vi "VISA LoopRead.vi"(8 "error in (no error)":errorcluster, 9 "byte count (350000)":u32=350000, 11 "VISA resource name":refnum<visa-resource-name>="GPIB0::4::INSTR") -> (0 "error out":errorcluster={"status"=FALSE, "code"=1073676294, "source"="VISA Read in CSA Measure.vi"}, 1 "Total Buffer":string, 3 "dup VISA resource name":refnum<visa-resource-name>="GPIB0::4::INSTR")   [LabVIEW 2011]
panel:
  out "Loops Performed":i32
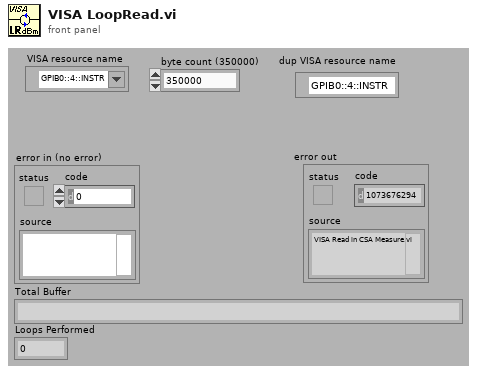
[diagram p1: front panel]
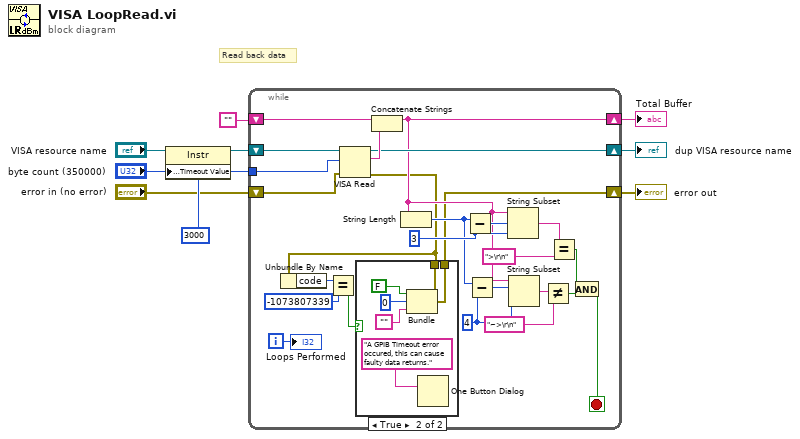
[diagram p0: block diagram]
diagram:
  # "Read back data"
  n1 = property class="Instr"(reference="VISA resource name", "General Settings:Timeout Value"=u32 3000) -> (reference out=w4:refnum<visa-resource-name>)  [unwired: 1 in, 1 out]
  n2 = while {
    shift-left: "error in (no error)" -> [w11]
    shift-right: [w17] -> w6
    shift-left: w4 -> [w10]
    shift-right: [w31] -> w7
    shift-left: "" -> [w32]
    shift-right: [w21] -> w8
    tunnel: "byte count (350000)" -> [w34]
    i -> [w15]
    stop <- w12 stop-if-true
    w22 = 4
    w29 = 3
    n3 = VISA Read(VISA resource name=w10, byte count=w34, error in (no error)=w11) -> (VISA resource name out=w31:refnum<visa-resource-name>, read buffer=w33:string, error out=w16:errorcluster)  [unwired: 1 out]
    n4 = Unbundle By Name(w16) -> ("code"=w19:i32)
    n5 = Equal?(x=w19, y=-1073807339) -> (x = y?=w20:bool)
    n6 = case shown="True" w20 {
      tunnel: [w35 w38] -> w17
      tunnel: w16 -> [w35 w37]
      frame False {
      }
      frame True {
        n7 = Bundle(cluster=w37, "status"=FALSE, "code"=0, "source"="") -> (w38:errorcluster)
        n8 = One Button Dialog(message="A GPIB Timeout error occured, this can cause faulty data returns.") -> ()  [unwired: 1 in, 1 out]
      }
    }
    n9 = Concatenate Strings(w32, w33) -> (w21:string)
    n10 = String Length(string=w21) -> (length=w24:i32)
    n11 = Subtract(x=w24, y=w29) -> (x-y=w30:i32)
    n12 = Subtract(x=w24, y=w22) -> (x-y=w23:i32)
    n13 = String Subset(string=w21, offset (0)=w30, length (rest)=w29) -> (substring=w28:string)
    n14 = String Subset(string=w21, offset (0)=w23, length (rest)=w22) -> (substring=w26:string)
    n15 = Not Equal?(x=w26, y="~>\r\n") -> (x != y?=w14:bool)
    n16 = Equal?(x=w28, y=">\r\n") -> (x = y?=w13:bool)
    n17 = And(x=w13, y=w14) -> (x .and. y?=w12:bool)
    "Loops Performed" <- w15
  }
  "dup VISA resource name" <- w7
  "error out" <- w6
  "Total Buffer" <- w8
